vi "EXT Trigger D1.vi"(8 "error in (no error)":errorcluster, 11 "VISA resource name":refnum<visa-resource-name>) -> (0 "value out":errorcluster, 3 "VISA resource name out":refnum<visa-resource-name>)   [LabVIEW 2025, in "Rigol.lvlib"]
uses:
  Rigol.lvlib
  954dfb8c-89f5-4d66-aae7-35f91b699eb2.vi
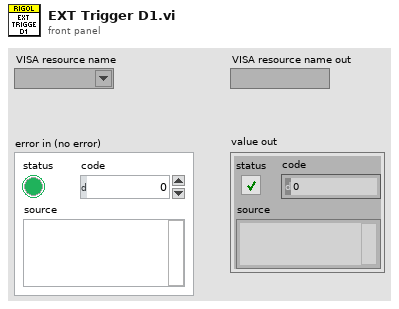
[diagram p1: front panel]
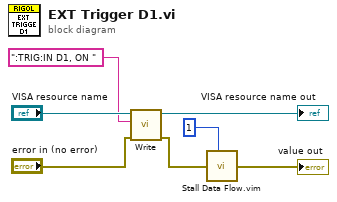
[diagram p0: block diagram]
diagram:
  n1 = call "Write.vi"("error in (no error)"="error in (no error)", "Write Buffer (\"\")"=":TRIG:IN D1, ON " ("format string"), "VISA resource name"="VISA resource name") -> ("error out"=w2:errorcluster, "VISA resource name out"=→"VISA resource name out":refnum<visa-resource-name>)  [unwired: 7 in]
  n2 = call "Stall Data Flow.vim"("value in"=w2, "milliseconds to wait"=u32 1) -> ("value out"=→"value out":errorcluster)  [unwired: 1 out]
